vi "Global 1.vi"() -> ()   [LabVIEW 2015]
panel:
  out "More Detection":T1(array[cluster])
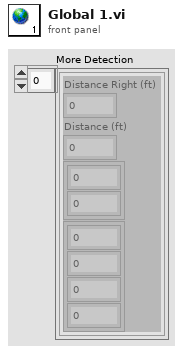
[diagram p1: front panel]
types:
  T1 = cluster{"Distance Right (ft)":dbl, "Distance (ft)":dbl, cluster{dbl, dbl}, cluster{dbl, dbl, dbl, dbl}}[]
diagram:
